vi "Worker Loop.vi"(11 "Worker Queue":refnum<queue>) -> ()   [LabVIEW 2016, in "Stream Log.lvlib" / "Asynchronous Application Log.lvclass"]
doc: "--\nCopyright © 2017 Composed SystemsI All rights reserved.\n\nAuthor: Jon McBee <jon.mcbee@composed.io>\n\nThis library is provided \"AS IS\" ,WITHOUT WARRANTIES OR\nCONDITIONS OF ANY KIND, either express or implied.\n\nComposed Systems -- composed.io\n\nStream 0.0.1.1\nJon McBee - Composed Systems\nCopyright (c) 2017, Composed Systems"
uses:
  <userlib>/Composed Systems/Stream/Log/Asynchronous Application Log/Asynchronous Application Log.lvclass
  <userlib>/Composed Systems/Stream/Log/Asynchronous Application Log/Message.ctl
  <userlib>/Composed Systems/Stream/Log/Asynchronous Application Log/Entry Type.ctl
  <userlib>/Composed Systems/Stream/Log/Log Sink/Log Sink.lvclass
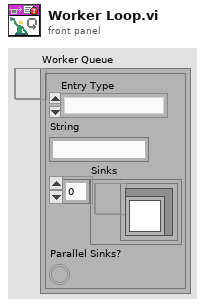
[diagram p1: front panel]
types:
  T1 = typedef "Stream Log.lvlib/Asynchronous Application Log.lvclass/Entry Type.ctl" = enum16{"Kill Worker", "Log Entry"}
  T2 = typedef "Stream Log.lvlib/Asynchronous Application Log.lvclass/Message.ctl" = cluster{"Entry Type":T1, "String":string, "Sinks":refnum<data-value>[], "Parallel Sinks?":bool}
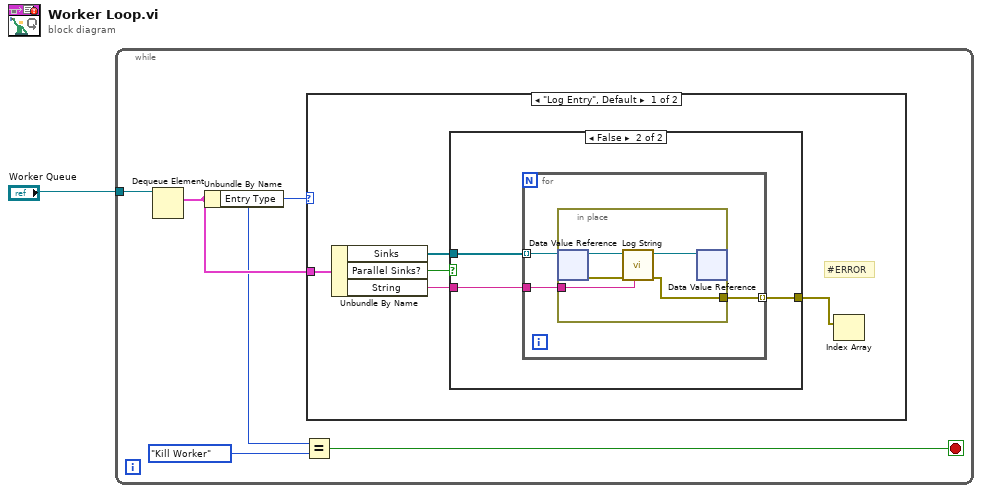
[diagram p0: block diagram]
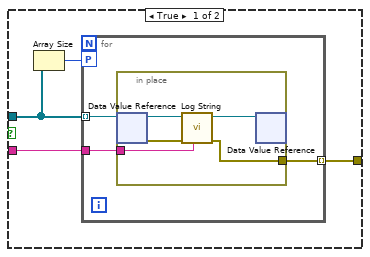
[diagram p2: hidden frame]
diagram:
  n1 = while {
    tunnel: "Worker Queue" -> [w6]
    stop <- w2 stop-if-true
    n2 = Dequeue Element(queue=w6) -> (element=w5:T2)  [unwired: 2 in, 3 out]
    n3 = Unbundle By Name(w5) -> ("Entry Type"=w4:T1)
    n4 = Equal?(x=w4, y=Entry_Type."Kill Worker") -> (x = y?=w2:bool)
    n5 = case shown="\"Log Entry\", Default" w4 {
      tunnel: w5 -> [w11 _]
      frame "Log Entry", Default {
        # "#ERROR"
        n6 = Unbundle By Name(w11) -> ("Sinks"=w9:refnum<data-value>[], "Parallel Sinks?"=w10:bool, "String"=w8:string)
        n7 = case shown="False" w10 {
          tunnel: w9 -> [w14 w26]
          tunnel: w8 -> [w13 w25]
          tunnel: [w12 w24] -> w7
          frame True {
            n8 = Array Size(array=w14) -> (size(s)=w15:i32)
            n9 = for {
              workers-P: w15 -> [_]
              tunnel: w14 -> [w18] mode=indexing
              tunnel: w13 -> [w17]
              tunnel: [w16] -> w12 mode=indexing
              n10 = in-place {
                in-place-border: w17 -> [w20]
                in-place-border: [w19] -> w16
                n11 = in-place-dvr #1(w18) -> (w23:refnum<class "Log Sink.lvclass">, w22:errorcluster)
                n12 = call-dynamic "Log String.vi"("String"=w20, "error in (no error)"=w22, "Log Sink in"=w23) -> ("error out"=w19:errorcluster, "Log Sink out"=w21:refnum<class "Log Sink.lvclass">)  [unwired: 7 in]
                n13 = in-place-dvr #1(w21) -> ()  [unwired: 2 out]
              }
            }
          }
          frame False {
            n14 = for {
              tunnel: w26 -> [w29] mode=indexing
              tunnel: w25 -> [w28]
              tunnel: [w27] -> w24 mode=indexing
              n15 = in-place {
                in-place-border: w28 -> [w31]
                in-place-border: [w30] -> w27
                n16 = in-place-dvr #2(w29) -> (w34:refnum<class "Log Sink.lvclass">, w33:errorcluster)
                n17 = call-dynamic "Log String.vi"("String"=w31, "error in (no error)"=w33, "Log Sink in"=w34) -> ("error out"=w30:errorcluster, "Log Sink out"=w32:refnum<class "Log Sink.lvclass">)  [unwired: 7 in]
                n18 = in-place-dvr #2(w32) -> ()  [unwired: 2 out]
              }
            }
          }
        }
        n19 = Index Array(array=w7) -> ()  [unwired: 1 in, 1 out]
      }
      frame "Kill Worker" {
      }
    }
  }
